vi "cmd获取计算机名.vi"() -> (2 "过滤后名":string, 3 "原名":string caption="计算机名")   [LabVIEW 2017]
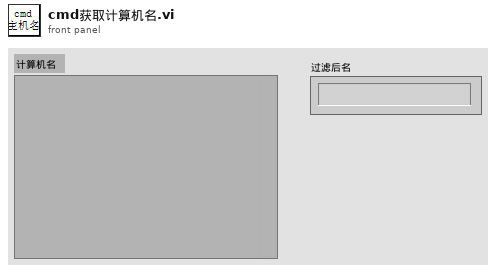
[diagram p1: front panel]
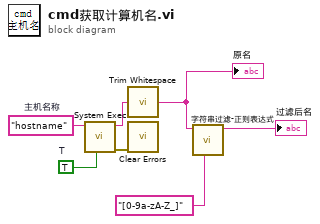
[diagram p0: block diagram]
diagram:
  w5 = TRUE  # T
  w7 = "hostname"  # 主机名称
  n1 = call <vilib>:"System Exec.vi"("run minimized? (F)"=w5, "command line"=w7) -> ("error out"=w4:errorcluster, "standard output"=w6:string)  [unwired: 6 in, 2 out]
  n2 = call <vilib>:"Trim Whitespace.vi"("string"=w6) -> ("trimmed string"=w3:string)  [unwired: 1 in]
  "原名" <- w3
  n3 = call <vilib>:"Clear Errors.vi"("error in (no error)"=w4) -> ()  [unwired: 5 in, 2 out]
  n4 = call "字符串过滤-正则表达式.vi"("正则式（非汉字单字符）"="[0-9a-zA-Z_]", "字符串 i"=w3) -> ("字符串 o"=→"过滤后名":string)  [unwired: 8 in, 1 out]
